vi "Set Save Object Dictionary.vi"(7 "timeout (1s)":dbl=1.0 min=0.0, 8 "error in (no error)":errorcluster, 11 "SDO object in":refnum<k20>) -> (0 "error out":errorcluster, 1 "completion code":u32, 3 "SDO object out":refnum<k20>)   [LabVIEW 2016]
uses:
  <vilib>/CANopenLib/CANOPEN.llb/CANopen SDO Write [STR].vi
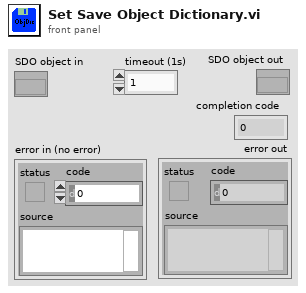
[diagram p1: front panel]
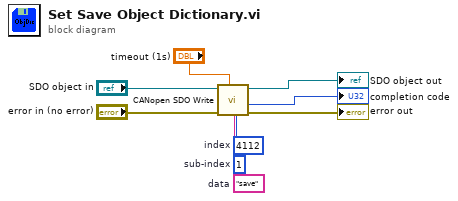
[diagram p0: block diagram]
diagram:
  w8 = "save"  # data
  w7 = u16 1  # sub-index
  w6 = u16 4112  # index
  n1 = call-poly <vilib>:"CANopen SDO Write.vi"("string data"=w8, "timeout (1s)"="timeout (1s)", "error in (no error)"="error in (no error)", "object sub-index (0)"=w7, "object index"=w6, "SDO object in"="SDO object in") -> ("error out"=→"error out":errorcluster, "completion code"=→"completion code":u32, "SDO object out"=→"SDO object out":refnum<k20>)  [unwired: 3 in]
